vi "LaunchChildren.vi"(8 "error in (no error)":errorcluster, 11 "TopLevel in":refnum<class "TopLevel.lvclass">) -> (0 "error out":errorcluster, 3 "TopLevel out":refnum<class "TopLevel.lvclass">)   [LabVIEW 2021, in "TopLevel.lvlib" / "TopLevel.lvclass"]
uses:
  TopLevel.lvclass
  C:/Program Files (x86)/National Instruments/LabVIEW 2021/vi.lib/ActorFramework/Actor/Actor.lvclass
  WebSocket/WebSocket/WebSocket.lvclass
  VisionUI/VisionUI/VisionUI.lvclass
  C:/Repos/Demo/Actors/Vision/Vision/Vision.lvclass
  TopLevel Messages/ReceiveCapturedImage Msg/ReceiveCapturedImage Msg.lvclass
  C:/Repos/Demo/Actors/Vision/Vision Messages/CapturedImage Msg/CapturedImage Msg.lvclass
  Vision/Vision/Vision.lvclass/Vision.ctl
  <vilib>/ActorFramework/Actor/Actor.lvclass
  Vision/Vision/Vision.lvclass
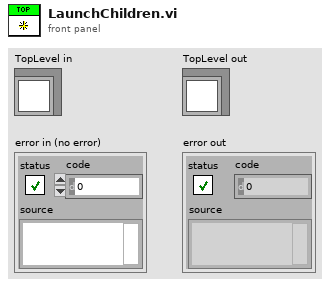
[diagram p1: front panel]
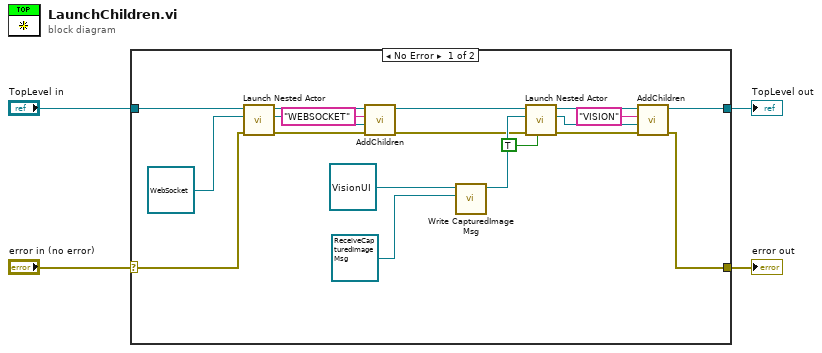
[diagram p0: block diagram]
diagram:
  n1 = case shown="No Error" "error in (no error)" {
    selector: "error in (no error)" -> [w15 w25]
    tunnel: [w6 w25] -> w3
    tunnel: [w8 w24] -> w1
    tunnel: "TopLevel in" -> [w23 w24]
    frame No Error {
      n2 = call <vilib>:"Launch Nested Actor.vi"("error in (no error)"=w15, "Nested Actor"=refnum<class "WebSocket.lvclass"> refnum ("WebSocket.lvlib:WebSocket.lvclass"), "Caller Actor in"=w23) -> ("error out"=w16:errorcluster, "Nested Actor's Enqueuer"=w17:refnum<class "Message Enqueuer.lvclass">, "Caller Actor out"=w19:refnum<class "TopLevel.lvclass">)  [unwired: 6 in]
      n3 = call "AddChildren.vi"("error in (no error)"=w16, "Enqueuer"=w17, "Actor Name"="WEBSOCKET", "TopLevel in"=w19) -> ("error out"=w10:errorcluster, "TopLevel out"=w14:refnum<class "TopLevel.lvclass">)  [unwired: 6 in]
      n4 = call "Write CapturedImage Msg.vi"("Vision.lvlib:CapturedImage Msg.lvclass"=refnum<class "ReceiveCapturedImage Msg.lvclass"> refnum ("TopLevel.lvlib:ReceiveCapturedImage Msg.lvclass"), "Vision in"=refnum<class "VisionUI.lvclass"> refnum ("VisionUI.lvlib:VisionUI.lvclass")) -> ("Vision out"=w13:refnum<class "VisionUI.lvclass">)  [unwired: 9 in]
      n5 = call <vilib>:"Launch Nested Actor.vi"("Open Actor Core front panel? (F)"=TRUE, "error in (no error)"=w10, "Nested Actor"=w13, "Caller Actor in"=w14) -> ("error out"=w11:errorcluster, "Nested Actor's Enqueuer"=w7:refnum<class "Message Enqueuer.lvclass">, "Caller Actor out"=w12:refnum<class "TopLevel.lvclass">)  [unwired: 5 in]
      n6 = call "AddChildren.vi"("error in (no error)"=w11, "Enqueuer"=w7, "Actor Name"="VISION", "TopLevel in"=w12) -> ("error out"=w6:errorcluster, "TopLevel out"=w8:refnum<class "TopLevel.lvclass">)  [unwired: 6 in]
    }
    frame Error {
    }
  }
  "error out" <- w3
  "TopLevel out" <- w1
